vi "Recurse.vi"(5 "Group Sizes":i32[](array[numeric]), 7 "Chars":string[](array[string]), 9 "Group Index":i32, 10 "Char Index":i32, 11 "Hash Count":i32) -> (3 "Number of aranagements":u64)   [LabVIEW 2021, in "Group.lvclass"]
uses:
  Group.lvclass
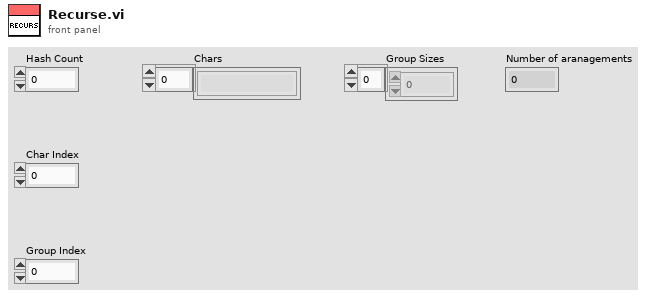
[diagram p1: front panel]
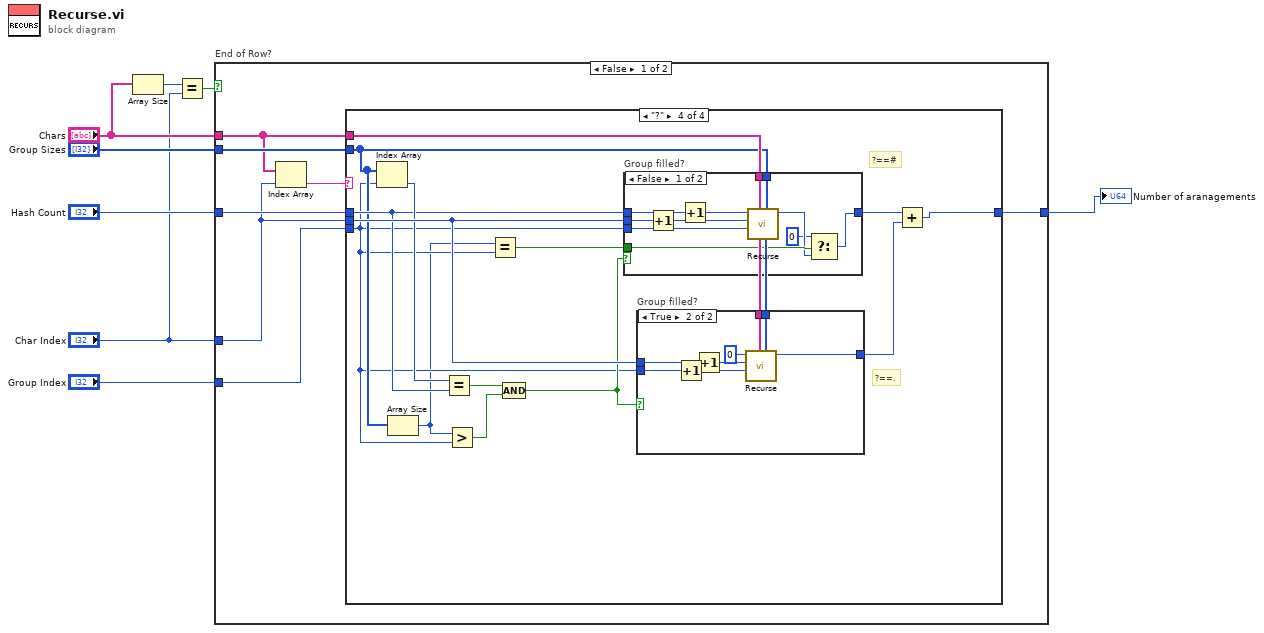
[diagram p0: block diagram]
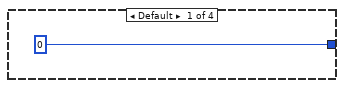
[diagram p2: hidden frame]
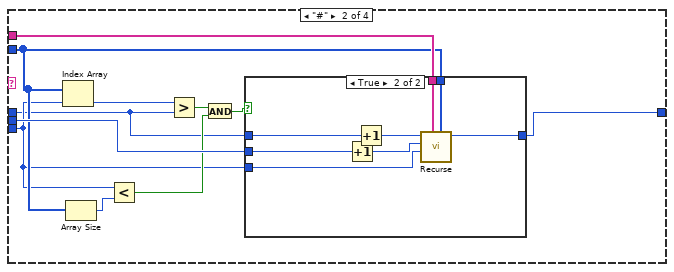
[diagram p3: hidden frame]
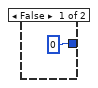
[diagram p4: hidden frame]
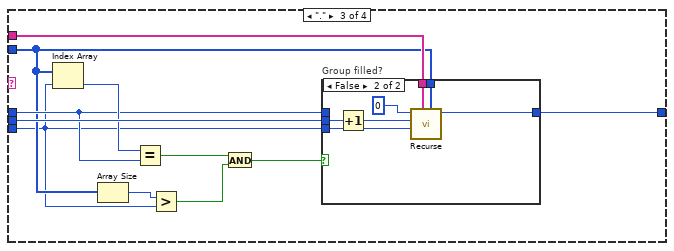
[diagram p5: hidden frame]
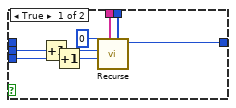
[diagram p6: hidden frame]
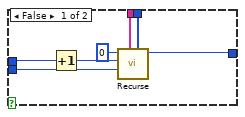
[diagram p7: hidden frame]
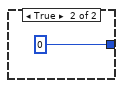
[diagram p8: hidden frame]
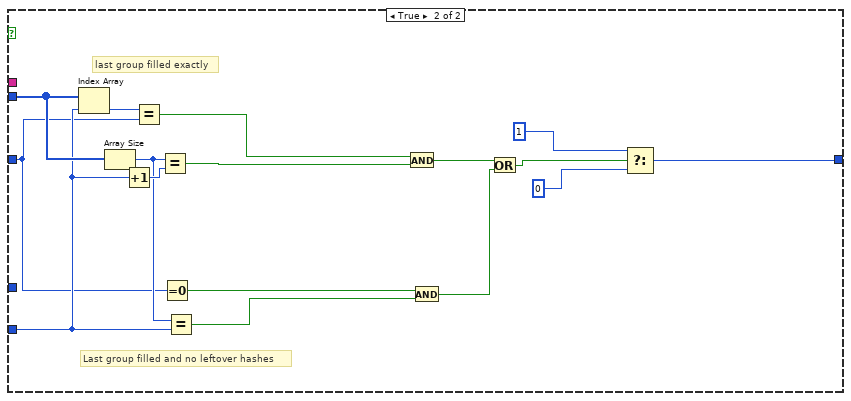
[diagram p9: hidden frame]
diagram:
  n1 = Array Size(array="Chars") -> (size(s)=w3:i32)
  n2 = Equal?(x=w3, y="Char Index") -> (x = y?=w1:bool)
  n3 = case "End of Row?" shown="False" w1 {
    tunnel: "Group Sizes" -> [w15 w113]
    tunnel: "Group Index" -> [w13 w109]
    tunnel: "Hash Count" -> [w12 w108]
    tunnel: [w11 w116] -> w5
    tunnel: "Chars" -> [w10 _]
    tunnel: "Char Index" -> [w9 _]
    frame False {
      n4 = Index Array(array=w10, index=w9) -> (element=w14:string)
      n5 = case shown="\"?\"" w14 {
        tunnel: w10 -> [_ w27 w47 w68]
        tunnel: w15 -> [_ w19 w41 w67]
        tunnel: w9 -> [_ w25 w46 w73]
        tunnel: w13 -> [_ w18 w39 w65]
        tunnel: w12 -> [_ w17 w43 w70]
        tunnel: [u64 0 ("Number of aranagements") w26 w45 w75] -> w11
        frame Default {
        }
        frame "#" {
          n6 = Index Array(array=w19, index=w18) -> (element=w20:i32)
          n7 = Array Size(array=w19) -> (size(s)=w23:i32)
          n8 = Less?(x=w18, y=w23) -> (x < y?=w21:bool)
          n9 = Greater?(x=w20, y=w17) -> (0:w24:bool)
          n10 = And(x=w24, y=w21) -> (x .and. y?=w22:bool)
          n11 = case shown="True" w22 {
            tunnel: w27 -> [_ w36]
            tunnel: w19 -> [_ w35]
            tunnel: [u64 0 ("Number of aranagements") w34] -> w26
            tunnel: w17 -> [_ w32]
            tunnel: w25 -> [_ w31]
            tunnel: w18 -> [_ w29]
            frame False {
            }
            frame True {
              n12 = Increment(x=w31) -> (x+1=w30:i32)
              n13 = Increment(x=w32) -> (x+1=w33:i32)
              n14 = call "Recurse.vi"("Group Sizes"=w35, "Chars"=w36, "Group Index"=w29, "Char Index"=w30, "Hash Count"=w33) -> ("Number of aranagements"=w34:u64)  [unwired: 6 in]
            }
          }
        }
        frame "." {
          n15 = Index Array(array=w41, index=w39) -> (element=w44:i32)
          n16 = Array Size(array=w41) -> (size(s)=w40:i32)
          n17 = Equal?(x=w44, y=w43) -> (x = y?=w42:bool)
          n18 = Greater?(x=w40, y=w39) -> (0:w37:bool)
          n19 = And(x=w42, y=w37) -> (x .and. y?=w38:bool)
          n20 = case "Group filled?" shown="False" w38 {
            tunnel: w47 -> [w55 w62]
            tunnel: w46 -> [w54 w61]
            tunnel: [w53 w60] -> w45
            tunnel: w41 -> [w52 w59]
            tunnel: w39 -> [w51 w58]
            tunnel: w43 -> [_ _]
            frame True {
              n21 = Increment(x=w54) -> (x+1=w49:i32)
              n22 = Increment(x=w51) -> (x+1=w50:i32)
              n23 = call "Recurse.vi"("Group Sizes"=w52, "Chars"=w55, "Group Index"=w50, "Char Index"=w49, "Hash Count"=0) -> ("Number of aranagements"=w53:u64)  [unwired: 6 in]
            }
            frame False {
              n24 = Increment(x=w61) -> (x+1=w57:i32)
              n25 = call "Recurse.vi"("Group Sizes"=w59, "Chars"=w62, "Group Index"=w58, "Char Index"=w57, "Hash Count"=0) -> ("Number of aranagements"=w60:u64)  [unwired: 6 in]
            }
          }
        }
        frame "?" {
          # "?==."
          # "?==#"
          n26 = Index Array(array=w67, index=w65) -> (element=w72:i32)
          n27 = Array Size(array=w67) -> (size(s)=w64:i32)
          n28 = Equal?(x=w72, y=w70) -> (x = y?=w71:bool)
          n29 = Greater?(x=w64, y=w65) -> (0:w69:bool)
          n30 = Equal?(x=w64, y=w65) -> (x = y?=w63:bool)
          n31 = Compound Arithmetic op=AND(w71, w69) -> (w66:bool)
          n32 = case "Group filled?" shown="False" w66 {
            tunnel: [w93 u64 0 ("Number of aranagements")] -> w76
            tunnel: w73 -> [w100 _]
            tunnel: w70 -> [w99 _]
            tunnel: w65 -> [w98 _]
            tunnel: w68 -> [w97 _]
            tunnel: w67 -> [w96 _]
            tunnel: w63 -> [w95 _]
            frame False {
              n33 = Increment(x=w100) -> (x+1=w101:i32)
              n34 = Increment(x=w99) -> (x+1=w102:i32)
              n35 = call "Recurse.vi"("Group Sizes"=w96, "Chars"=w97, "Group Index"=w98, "Char Index"=w101, "Hash Count"=w102) -> ("Number of aranagements"=w94:u64)  [unwired: 6 in]
              n36 = Select(t=u64 0 ("f"), s=w95, f=w94) -> (s? t:f=w93:u64)
            }
            frame True {
            }
          }
          n37 = case "Group filled?" shown="True" w66 {
            tunnel: [w81 w91] -> w74
            tunnel: w73 -> [w79 w90]
            tunnel: w65 -> [w78 w89]
            tunnel: w68 -> [w83 w88]
            tunnel: w67 -> [w82 w87]
            frame False {
              n38 = Increment(x=w79) -> (x+1=w77:i32)
              n39 = call "Recurse.vi"("Group Sizes"=w82, "Chars"=w83, "Group Index"=w78, "Char Index"=w77, "Hash Count"=0) -> ("Number of aranagements"=w81:u64)  [unwired: 6 in]
            }
            frame True {
              n40 = Increment(x=w89) -> (x+1=w86:i32)
              n41 = Increment(x=w90) -> (x+1=w85:i32)
              n42 = call "Recurse.vi"("Group Sizes"=w87, "Chars"=w88, "Group Index"=w86, "Char Index"=w85, "Hash Count"=0) -> ("Number of aranagements"=w91:u64)  [unwired: 6 in]
            }
          }
          n43 = Add(x=w76, y=w74) -> (x+y=w75:u64)
        }
      }
    }
    frame True {
      # "Last group filled and no leftover hashes"
      # "last group filled exactly"
      n44 = Index Array(array=w113, index=w109) -> (element=w119:i32)
      n45 = Array Size(array=w113) -> (size(s)=w110:i32)
      n46 = Increment(x=w109) -> (x+1=w112:i32)
      n47 = Equal?(x=w119, y=w108) -> (x = y?=w118:bool)
      n48 = Equal?(x=w110, y=w112) -> (x = y?=w114:bool)
      n49 = Equal To 0?(x=w108) -> (x = 0?=w107:bool)
      n50 = Equal?(x=w110, y=w109) -> (x = y?=w106:bool)
      n51 = And(x=w118, y=w114) -> (x .and. y?=w115:bool)
      n52 = And(x=w107, y=w106) -> (x .and. y?=w104:bool)
      n53 = Or(x=w115, y=w104) -> (x .or. y?=w105:bool)
      n54 = Select(t=u64 1 ("Number of aranagements"), s=w105, f=u64 0) -> (s? t:f=w116:u64)
    }
  }
  "Number of aranagements" <- w5
